vi "N4_201_write_range.vi"(0 "DriverConnect in":T1={"InterfaceType"=enum."VISA", "OpenedSession"="", "InterfaceSettings"={"Interface"=enum."RS232", "EOS 4 read"=enum."LF (\\n)", "EOS 4 write"=enum."LF (\\n)", "TMO, ms"=10000, "Sett"=variant(cluster{"Baud Rate":u32, "Data Bits":u16, "Parity":u16, "Stop Bits":u16, "Flow Control":u16, "Eho":bool} {"Baud Rate"=75, "Data Bits"=0, "Parity"=0, "Stop Bits"=0, "Flow Control"=0, "Eho"=FALSE})}}, 1 "Command range":T7, 2 "ModeIsChanged?":T6, 11 "error in":T8, 12 "Error Code":T10, 13 "Command mode":T7, 14 "Driver Name":T9) -> (4 "DriverConnect out":T1={"InterfaceType"=enum."VISA", "OpenedSession"="", "InterfaceSettings"={"Interface"=enum."RS232", "EOS 4 read"=enum."LF (\\n)", "EOS 4 write"=enum."LF (\\n)", "TMO, ms"=10000, "Sett"=variant(cluster{"Baud Rate":u32, "Data Bits":u16, "Parity":u16, "Stop Bits":u16, "Flow Control":u16, "Eho":bool} {"Baud Rate"=75, "Data Bits"=0, "Parity"=0, "Stop Bits"=0, "Flow Control"=0, "Eho"=FALSE})}}, 8 "RangeWasChanged":T6=TRUE, 15 "error out":T8)   [LabVIEW 2018]
uses:
  MOKO_LabViewLibrary/MokoLowLevel/MokoLowLovelControl/MLLC_ErrorCode.ctl
  MOKO_LabViewLibrary/MokoLowLevel/MokoLowLovelControl/MLLC_DriverName.ctl
  MOKO_LabViewLibrary/MokoLowLevel/MokoLowLovelControl/MLLC_Error.ctl
  MOKO_LabViewLibrary/MokoLowLevel/MokoLowLovelControl/MLLC_Command.ctl
  MOKO_LabViewLibrary/MokoLowLevel/MokoLowLovelControl/MLLC_Boolean.ctl
  MOKO_LabViewLibrary/MokoLowLevel/MokoLowLovelControl/MLLC_DriverConnectCluster.ctl
  MOKO_LabViewLibrary/MokoLowLevel/MokoLowLovelControl/MLLC_InterfaceType.ctl
  MOKO_LabViewLibrary/MokoLowLevel/MokoLowLovelControl/MLLC_OpenedSession.ctl
  MOKO_LabViewLibrary/MokoLowLevel/MokoLowLovelControl/MLLC_InterfaceSettings.ctl
  MOKO_LabViewLibrary/MokoLowLevel/MokoLowLovelControl/MLLC_InterfaceKind.ctl
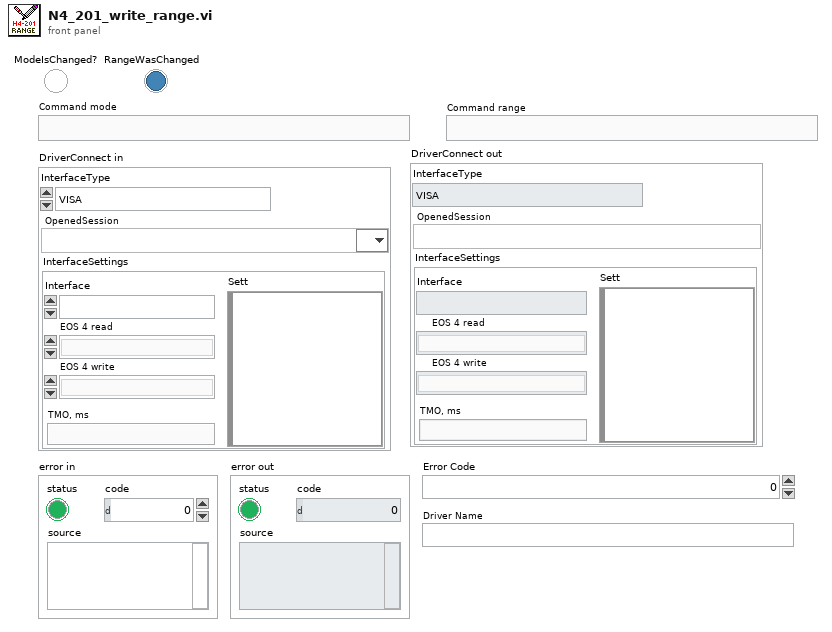
[diagram p1: front panel]
types:
  T1 = typedef "MLLC_DriverConnectCluster.ctl" = cluster{"InterfaceType":T2, "OpenedSession":T3, "InterfaceSettings":T4}
  T2 = typedef "MLLC_InterfaceType.ctl" = enum16{"VISA", "Prologix USB-GPIB"}
  T3 = typedef "MLLC_OpenedSession.ctl" = refnum<visa-resource-name>
  T4 = typedef "MLLC_InterfaceSettings.ctl" = cluster{"Interface":T5, "EOS 4 read":enum16{"Default (=EOS 4 write)", "CR (\\r)", "LF (\\n)", "None"}, "EOS 4 write":enum16{"CR+LF (\\r\\n)", "CR (\\r)", "LF (\\n)", "None"}, "TMO, ms":i32, "Sett":variant}
  T5 = typedef "MLLC_InterfaceKind.ctl" = enum16{"RS232", "GPIB", "USB", "Ethernet", "another"}
  T6 = typedef "MLLC_Boolean.ctl" = bool
  T7 = typedef "MLLC_Command.ctl" = string
  T8 = typedef "MLLC_Error.ctl" = errorcluster
  T9 = typedef "MLLC_DriverName.ctl" = string
  T10 = typedef "MLLC_ErrorCode.ctl" = u32
  T11 = enum16{"Нет симуляции", "В ручную", "Игнорировать"}
  T12 = typedef "MLLC_Response.ctl" = string
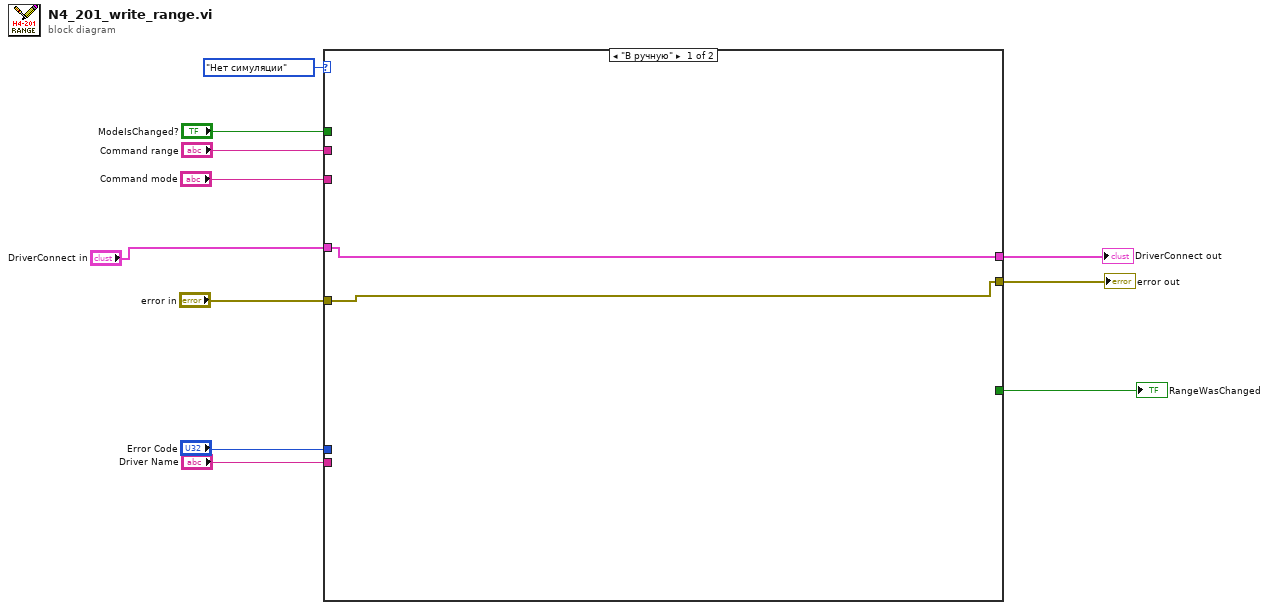
[diagram p0: block diagram]
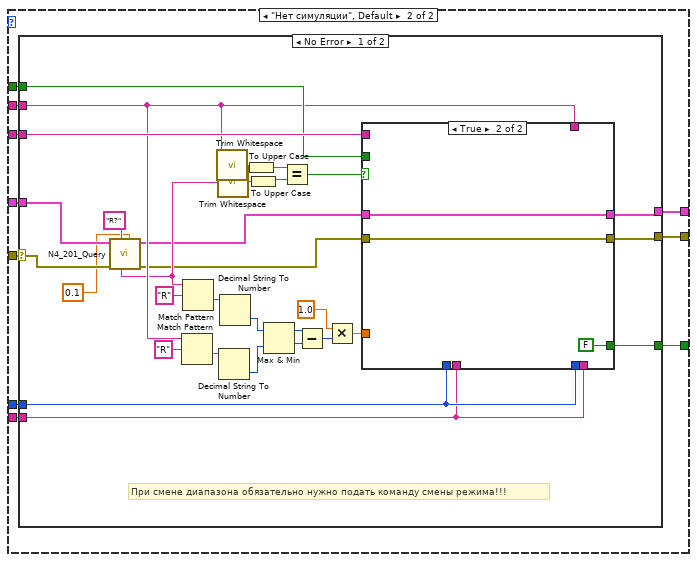
[diagram p2: hidden frame]
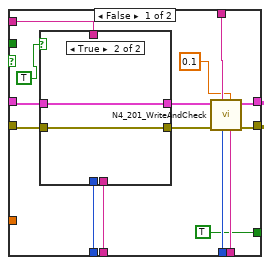
[diagram p3: hidden frame]
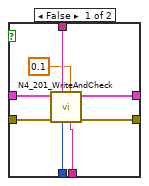
[diagram p4: hidden frame]
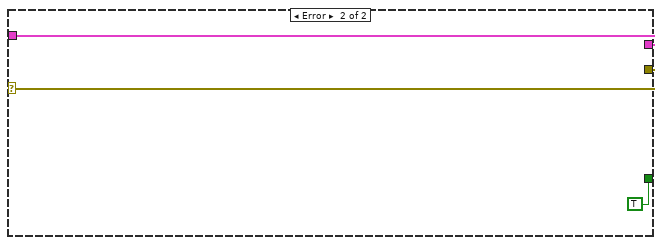
[diagram p5: hidden frame]
diagram:
  n1 = case shown="\"В ручную\"" T11."Нет симуляции" ("Simmulation") {
    tunnel: [w12 w23] -> w11
    tunnel: "Error Code" -> [_ w22]
    tunnel: "Driver Name" -> [_ w21]
    tunnel: "DriverConnect in" -> [w13 w20]
    tunnel: "error in" -> [w12 w19]
    tunnel: "Command range" -> [_ w18]
    tunnel: [w13 w17] -> w1
    tunnel: "Command mode" -> [_ w16]
    tunnel: [_ w15] -> w5
    tunnel: "ModeIsChanged?" -> [_ w14]
    frame "В ручную" {
    }
    frame "Нет симуляции", Default {
      n2 = case shown="No Error" w19 {
        selector: w19 -> [w49 w85]
        tunnel: [w52 w85] -> w23
        tunnel: [w53 w84] -> w17
        tunnel: w22 -> [w48 _]
        tunnel: w21 -> [w47 _]
        tunnel: w20 -> [w54 w84]
        tunnel: w18 -> [w45 _]
        tunnel: w16 -> [w50 _]
        tunnel: [w51 TRUE] -> w15
        tunnel: w14 -> [w46 _]
        frame No Error {
          # "При смене диапазона обязательно нужно подать команду смены режима!!!"
          n3 = call "N4_201_Query.vi"("Delay Befor (s)"=0.1 ("Command Time (s)"), "Command"="R?" ("Error Query"), "error in"=w49, "DriverConnect in"=w54) -> ("error out"=w25:T8, "DriverConnect out"=w26:T1, "Response"=w27:T12)  [unwired: 5 in]
          n4 = Match Pattern(string=w45, regular expression="R") -> (after substring=w36:T7)  [unwired: 1 in, 3 out]
          n5 = Match Pattern(string=w27, regular expression="R") -> (after substring=w37:T12)  [unwired: 1 in, 3 out]
          n6 = call <vilib>:"Trim Whitespace.vi"("string"=w45) -> ("trimmed string"=w40:string)  [unwired: 1 in]
          n7 = call <vilib>:"Trim Whitespace.vi"("string"=w27) -> ("trimmed string"=w42:string)  [unwired: 1 in]
          n8 = Decimal String To Number(string=w36) -> (number=w33:i32)  [unwired: 2 in, 1 out]
          n9 = Decimal String To Number(string=w37) -> (number=w34:i32)  [unwired: 2 in, 1 out]
          n10 = To Upper Case(1:w40) -> (0:w41:string)
          n11 = To Upper Case(1:w42) -> (0:w43:string)
          n12 = Max & Min(x=w34, y=w33) -> (max(x,y)=w32:i32, min(x,y)=w31:i32)
          n13 = Equal?(x=w41, y=w43) -> (x = y?=w39:bool)
          n14 = Subtract(x=w32, y=w31) -> (x-y=w30:i32)
          n15 = Multiply(x=1.0 ("Delay Time (s)"), y=w30) -> (x*y=w29:dbl)
          n16 = case shown="True" w39 {
            tunnel: w48 -> [w69 _]
            tunnel: w47 -> [w68 _]
            tunnel: [w67 w82] -> w53
            tunnel: [w66 w81] -> w52
            tunnel: w45 -> [w65 _]
            tunnel: w26 -> [w63 w82]
            tunnel: w25 -> [w57 w81]
            tunnel: [TRUE FALSE] -> w51
            tunnel: w50 -> [w62 _]
            tunnel: w48 -> [w61 _]
            tunnel: w47 -> [w60 _]
            tunnel: w46 -> [_ _]
            tunnel: w29 -> [_ _]
            frame False {
              n17 = case shown="True" TRUE {
                tunnel: w63 -> [w77 w79]
                tunnel: w62 -> [w76 _]
                tunnel: w61 -> [w75 _]
                tunnel: w60 -> [w74 _]
                tunnel: [w73 w79] -> w59
                tunnel: [w72 w78] -> w58
                tunnel: w57 -> [w71 w78]
                frame False {
                  n18 = call "N4_201_WriteAndCheck.vi"("Driver Name"=w74, "Command Time (s)"=0.1 ("Delay Time (s)"), "Error Code"=w75, "Command"=w76, "error in"=w71, "DriverConnect in"=w77) -> ("error out"=w72:T8, "DriverConnect out"=w73:T1)  [unwired: 4 in]
                }
                frame True {
                }
              }
              n19 = call "N4_201_WriteAndCheck.vi"("Driver Name"=w68, "Command Time (s)"=0.1, "Error Code"=w69, "Command"=w65, "error in"=w58, "DriverConnect in"=w59) -> ("error out"=w66:T8, "DriverConnect out"=w67:T1)  [unwired: 4 in]
            }
            frame True {
            }
          }
        }
        frame Error {
        }
      }
    }
  }
  "error out" <- w11
  "RangeWasChanged" <- w5
  "DriverConnect out" <- w1
